vi "try_Listbox Row Options.vi"() -> ()   [LabVIEW 2025]
panel:
  in  "Alternate Row Background Color":u32(colorbox)=13497576
  in  "Stop":bool
  in  "Word Wrapping":bool
  in  "Alternate Row Colors":bool
  in  "US Presidents":i32(listbox)
  # "Scenario\nListboxes, Trees, and Tables now support the ability to display alternating row background colors. Additionally, they support the ability to word wrap row contents\n\nInstructions\n1. To display alternate row background colors right click the US Presidents Listbox>>Row Options>>Alternating Colors \n2. To word wrap row contents right click the US Presidents Listbox>>Row Options>>Word Wrap\n3. Alternatively enable and disable these properties programatically. For this Run the VI and use the Alternate Row Colors and Word Wrapping switches"
  # "Off"
  # "On"
  # "Off"
  # "On"
  # "Close this VI when you are done with the demo."
  # "You do not need to save changes to this VI."
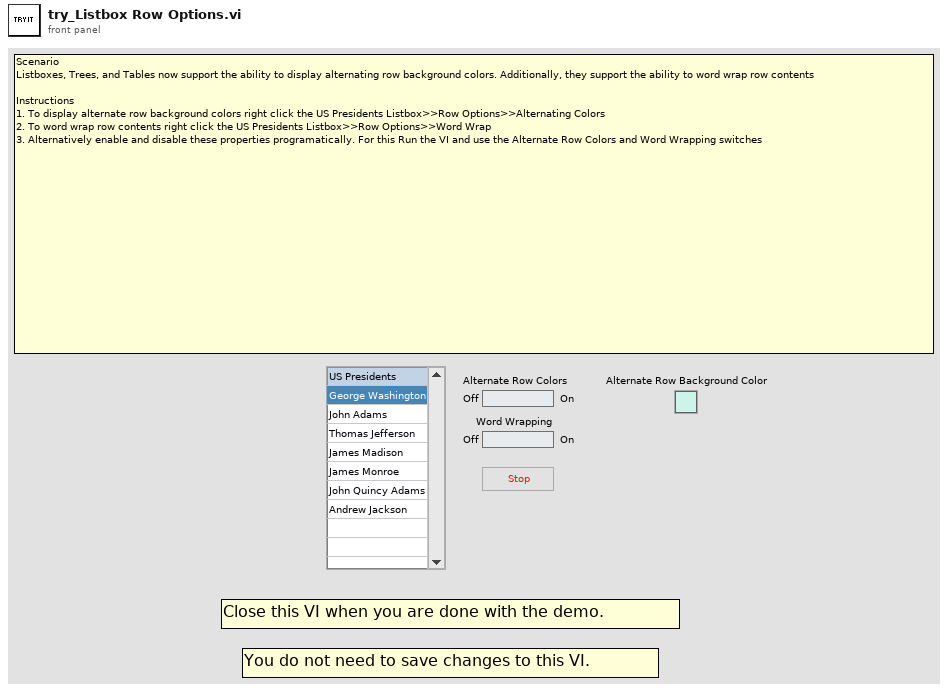
[diagram p1: front panel]
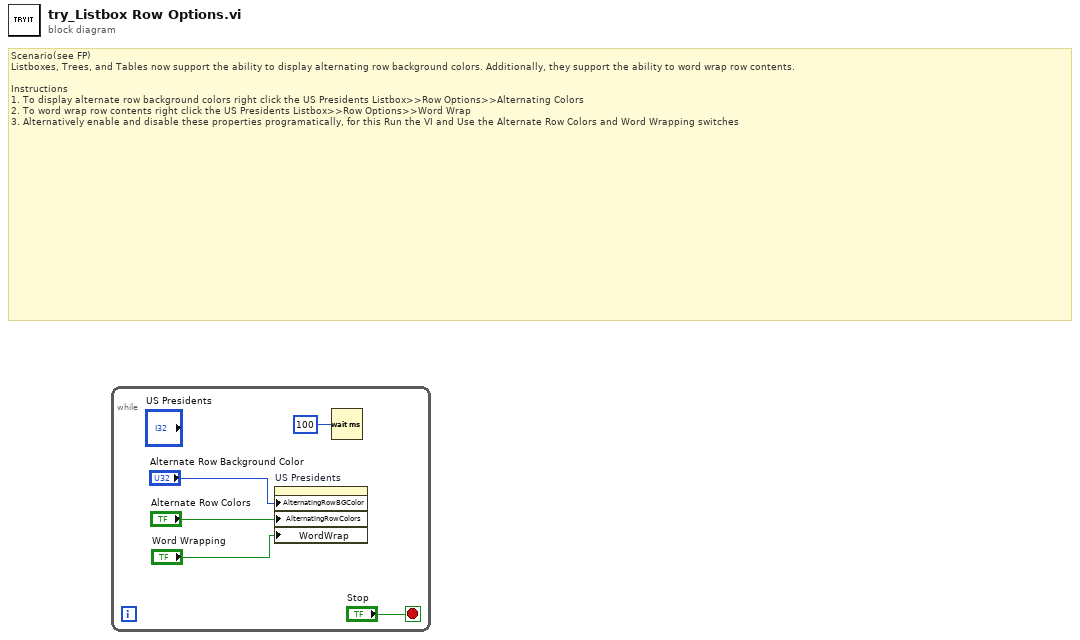
[diagram p0: block diagram]
diagram:
  # "Scenario(see FP)\nListboxes, Trees, and Tables now support the ability to display alternating row background colors. Additionally, they support the ability to word wrap row contents.\n\nInstructions\n1. To display alternate row background colors right click the US Presidents Listbox>>Row Options>>Alternating Colors \n2. To word wrap row contents right click the US Presidents Listbox>>Row Options>>Word Wrap\n3. Alternatively enable and disable these properties programatically, for this Run the VI and Use the Alternate Row Colors and Word Wrapping switches"
  n1 = while {
    stop <- "Stop" stop-if-true
    n2 = property on="US Presidents" class="LstBox (strict)"("AlternatingRowBGColor"="Alternate Row Background Color", "AlternatingRowColors"="Alternate Row Colors", "WordWrap"="Word Wrapping") -> ()  [unwired: 2 in, 2 out]
    n3 = Wait (ms)(milliseconds to wait=u32 100) -> ()  [unwired: 1 out]
  }
